vi "Enqueue Message.vi"(8 "error in (no error)":errorcluster, 9 "Message Data":variant, 10 "Message":string, 11 "Process In":refnum<class "Process.lvclass">) -> (0 "error out":errorcluster, 3 "Process Out":refnum<class "Process.lvclass">)   [LabVIEW 2020, in "Process.lvclass"]
doc: "Enqueue a message to the process. The message is received and should be handled in the Handle Messages VI."
uses:
  Process.lvclass
  Process.lvclass/Process.ctl
  Message Cluster.ctl
  Request Message Cluster.ctl
  <vilib>/Utility/error.llb/Clear Errors.vi
  <vilib>/Utility/error.llb/Error Cluster From Error Code.vi
  <vilib>/ErrorRing/Error Ring.xnode
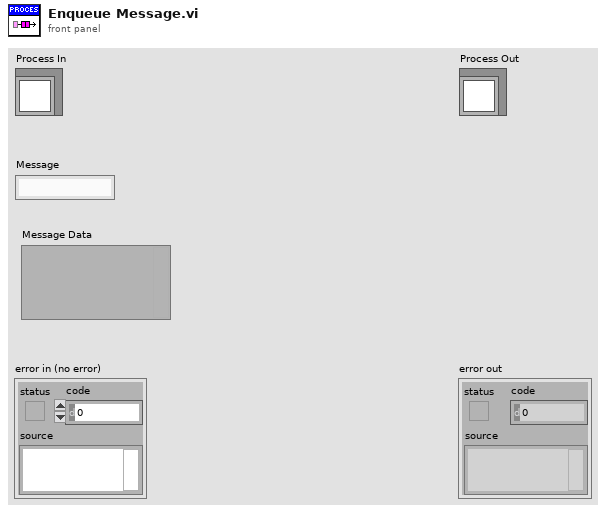
[diagram p1: front panel]
types:
  T1 = typedef "Process.lvclass/Message Cluster.ctl" = cluster{"Message":string, "Message Data":variant, "Request Notifier":refnum<notifier>}
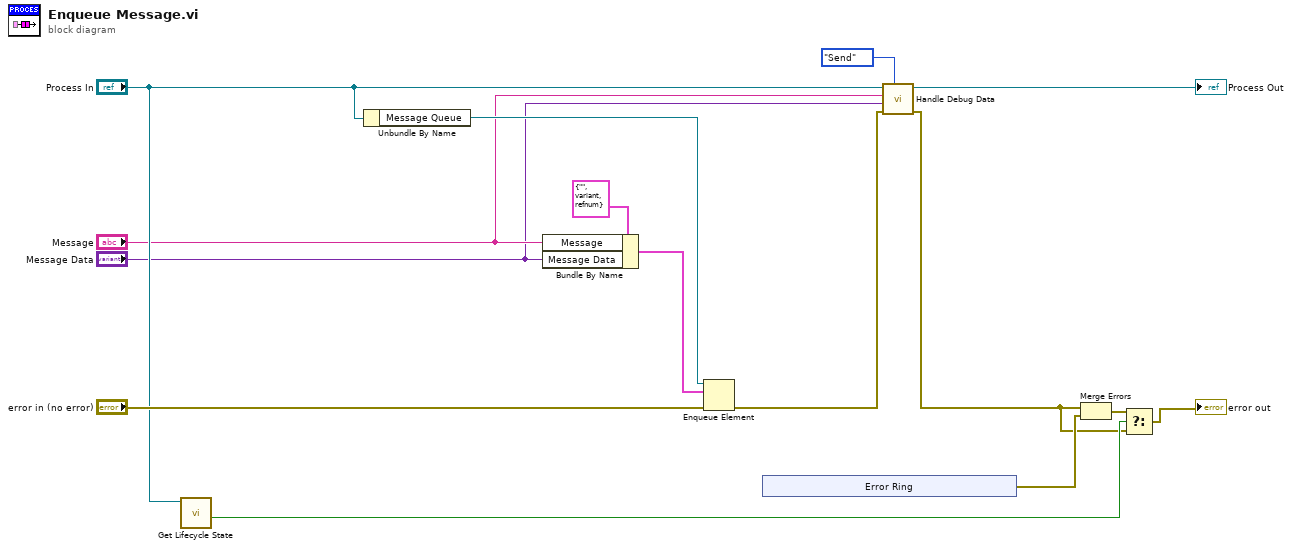
[diagram p0: block diagram]
diagram:
  n1 = call "Get Lifecycle State.vi"("Process In"="Process In") -> ("In Process Loop?"=w11:bool)  [unwired: 7 in, 3 out]
  n2 = Unbundle By Name("Process In") -> ("Message Queue"=w8:refnum<queue>)
  n3 = Bundle By Name(cluster=T1 {"Message"="", "Message Data"=variant, "Request Notifier"=refnum} ("Message Cluster"), "Message"="Message", "Message Data"="Message Data") -> (w7:T1)
  n4 = Enqueue Element(queue=w8, element=w7, error in (no error)="error in (no error)") -> (error out=w5:errorcluster)  [unwired: 1 in, 2 out]
  n5 = xnode "Error Ring"() -> ("error out"=w9:errorcluster)
  n6 = call "Handle Debug Data.vi"("Action"=enum16{"Send", "Receive", "Request", "Response"}."Send", "error in (no error)"=w5, "Message Data"="Message Data", "Message"="Message", "Process In"="Process In") -> ("error out"=w4:errorcluster, "Process Out"=→"Process Out":refnum<class "Process.lvclass">)  [unwired: 5 in]
  n7 = Merge Errors(w4, w9) -> (w10:errorcluster)
  n8 = Select(t=w10, s=w11, f=w4) -> (s? t:f=→"error out":errorcluster)
